vi "Wave2D_Solve UPT.vi"(9 "LU of P":T1, 10 "P":T3, 11 "U":dbl[][](array[numeric])) -> (0 "error":i32, 3 "U/PT":dbl[][](array[numeric]))   [LabVIEW 2017, in "NI_PDE.lvlib"]
uses:
  <vilib>/gmath/NI_PDE.lvlib
  <vilib>/Analysis/Matrix/Datatypes/RealMatrix.ctl
  <vilib>/Analysis/Matrix/NI_Matrix.lvlib
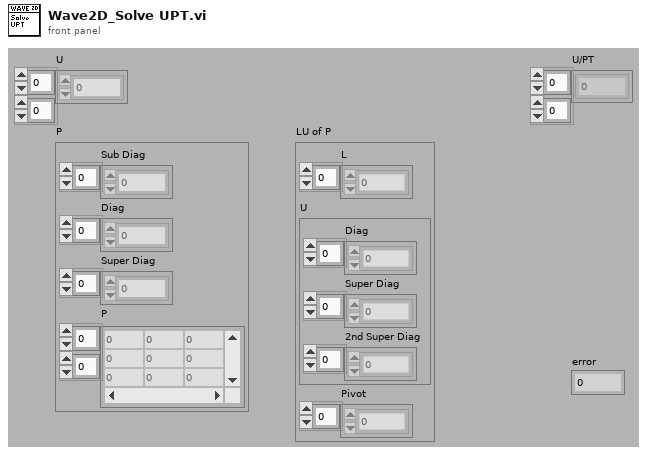
[diagram p1: front panel]
types:
  T1 = cluster{"L":dbl[], "U":cluster{"Diag":dbl[], "Super Diag":dbl[], "2nd Super Diag":dbl[]}, "Pivot":i32[]}
  T2 = typedef "NI_Matrix.lvlib/RealMatrix.ctl" = dbl[][]
  T3 = cluster{"Sub Diag":dbl[], "Diag":dbl[], "Super Diag":dbl[], "P":T2}
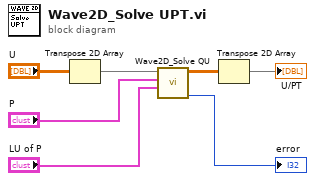
[diagram p0: block diagram]
diagram:
  n1 = Transpose 2D Array(2D array="U") -> (transposed array=w3:dbl[][])
  n2 = call <vilib>:"Wave2D_Solve QU.vi"("LU of Q"="LU of P", "Q"="P", "U"=w3) -> ("error"=→"error":i32, "Q\\U"=w2:dbl[][])  [unwired: 7 out]
  n3 = Transpose 2D Array(2D array=w2) -> (transposed array=→"U/PT":dbl[][])
